vi "VgSweep_TdepRoshan.vi"() -> ()   [LabVIEW 2013]
panel:
  out "Experiment ends at:":string
  in  "How many\npoints:":i16=10 min=-4 max=4 step=1
  in  "Step (K):":dbl=10.0 min=-4.0 max=4.0 step=1.0
  in  "T dependence:":T1(radio)
  in  "Optional custom folder":string
  out "Sweep":i16
  out "T Array":dbl[](array[numeric])
  out "minutes":dbl caption="Last full sweep took:" format="%#.1g"
  in  "Faster":dbl=10.0
  in  "HigherRate?":bool
  out "Current T (K)":dbl min=-4.0 max=4.0 step=0.1 format="%.2f"
  out "T-control\nGPIB":string="24"
  out "Hours":dbl format="%.1f"
  in  "Start sweeping":bool
  out "Of":i16
  out "Estimated time of experiment:":i16
  in  "Sweeps at each T:":i16=1 min=-4 max=4 step=1
  in  "Final T (K)":dbl=145.0 min=-4.0 max=4.0 step=0.1 format="%.2f"
  in  "Initial T (K)":dbl=125.0 min=-4.0 max=4.0 step=0.1 format="%.2f"
  in  "V2:":dbl=1.0 min=-4.0 max=4.0 step=0.1 format="%.3f"
  in  "Sweep rate , V/min":dbl=0.6 min=0.0 max=1.0 step=0.01 format="%.4f"
  in  "V1:":dbl min=-4.0 max=4.0 step=0.1 format="%.3f"
  # "Define interval of gate voltage\nfor main Keithley 2400 (address 12):"
  # "Set temperatures at which sweeps\nare made"
  # "min."
  # "="
  # "hours"
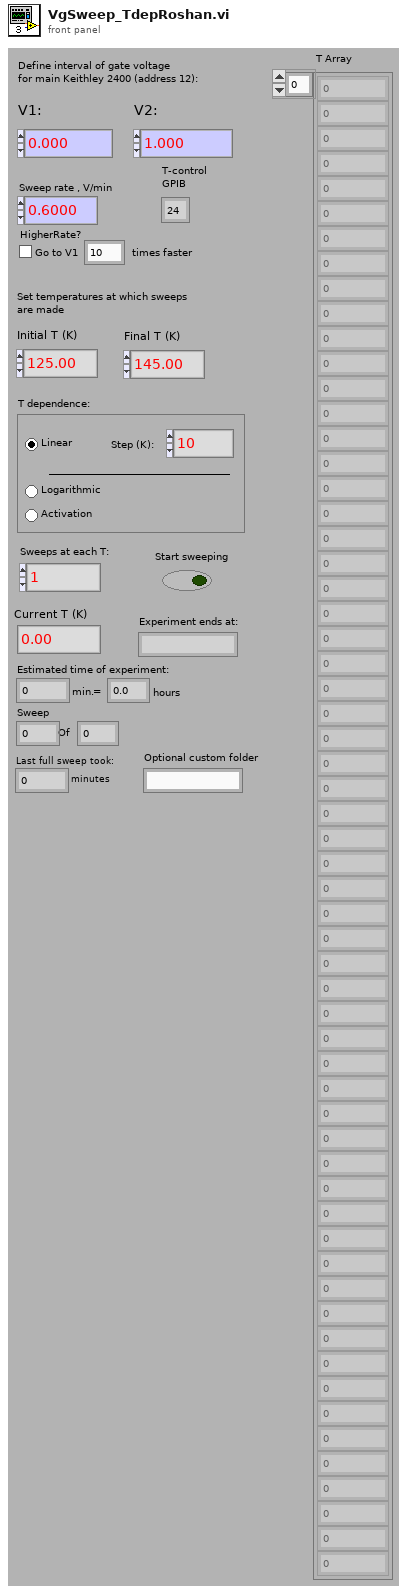
[diagram p1: front panel]
types:
  T1 = enum32{"Radio Selection 1", "Radio Selection 2", "Radio Selection 3"}
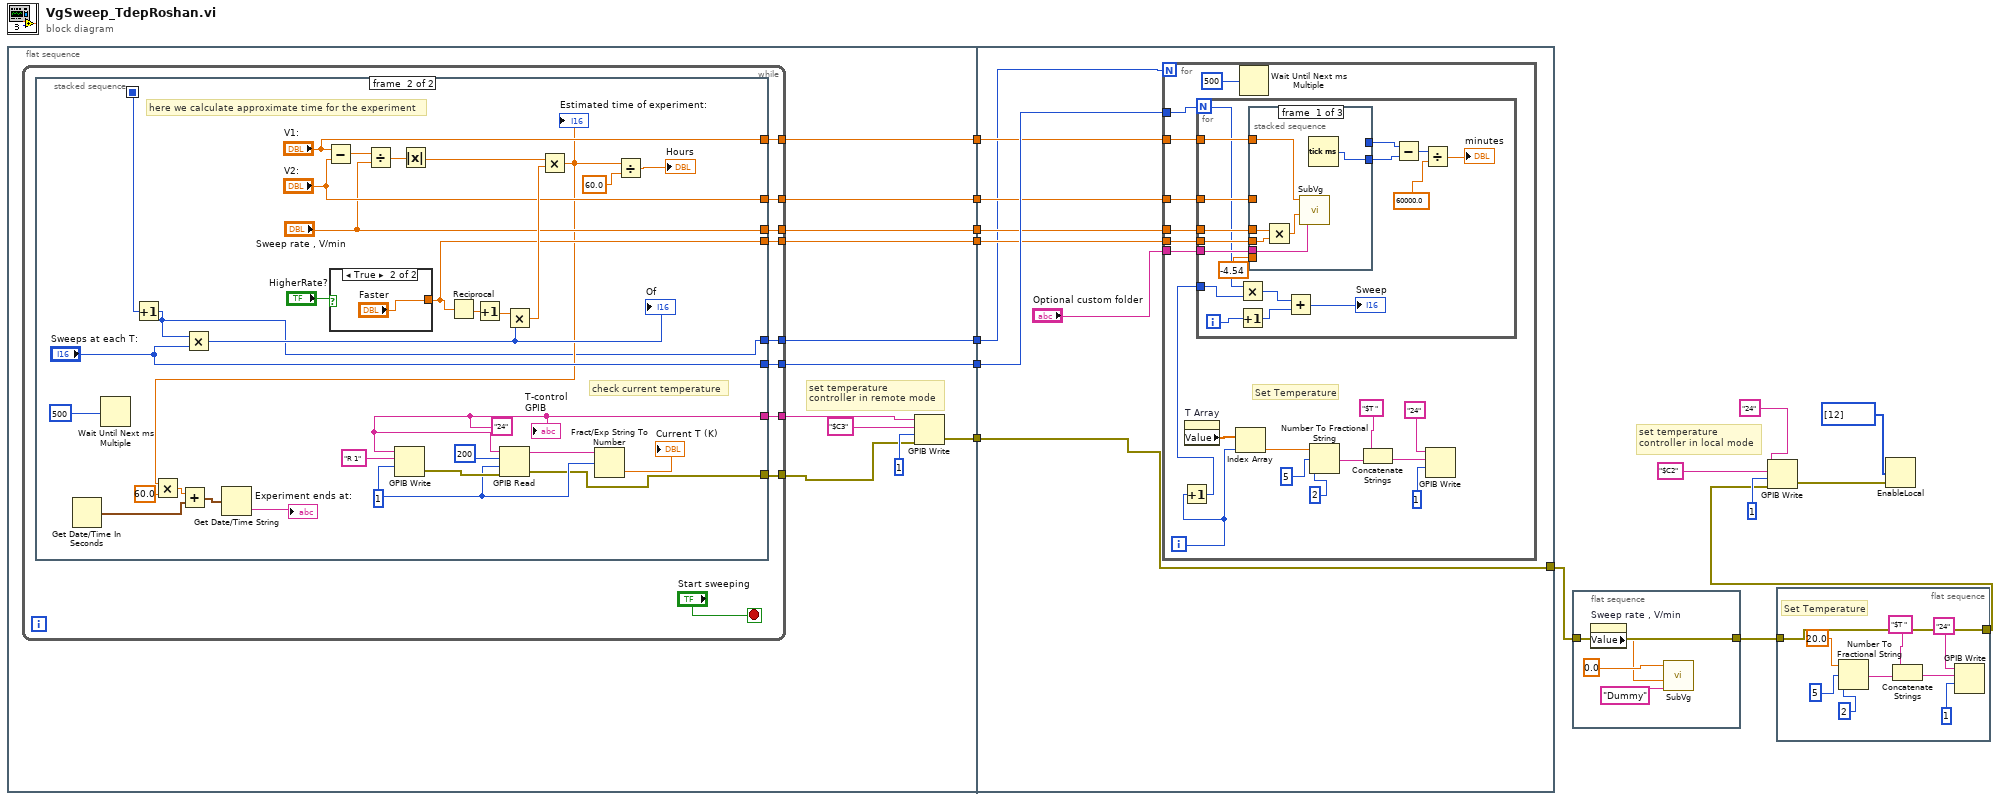
[diagram p0: block diagram]
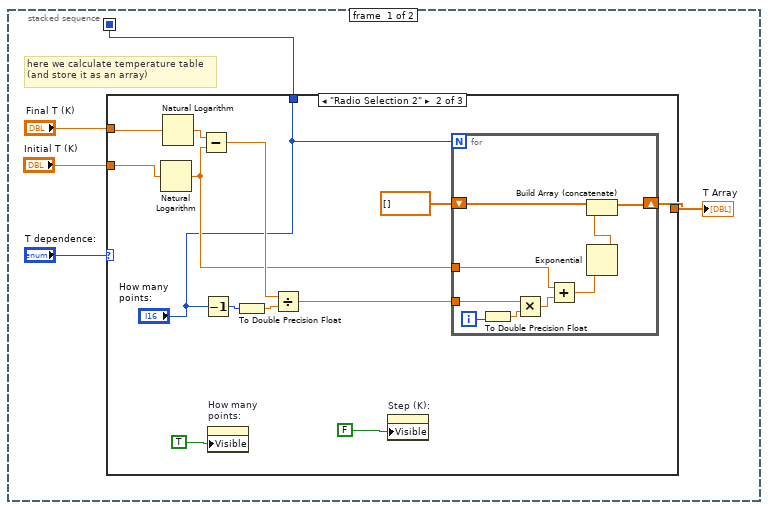
[diagram p2: hidden frame]
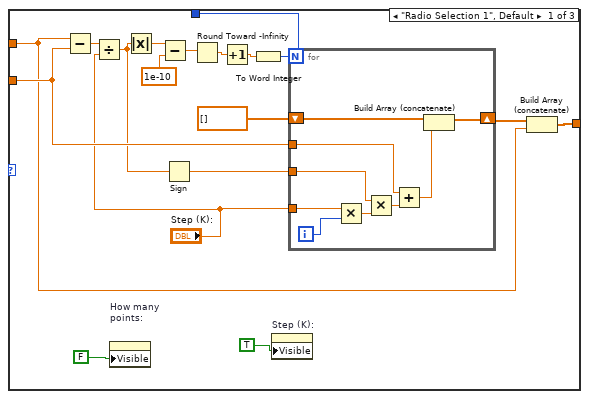
[diagram p3: hidden frame]
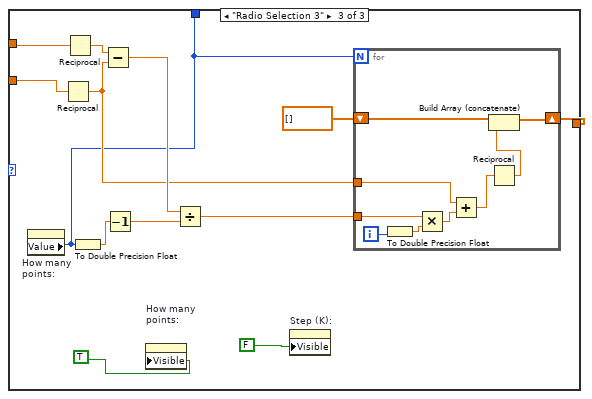
[diagram p4: hidden frame]
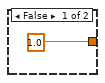
[diagram p5: hidden frame]
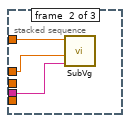
[diagram p6: hidden frame]
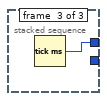
[diagram p7: hidden frame]
diagram:
  # "set temperature\ncontroller in local mode"
  n1 = flat-sequence {
    tunnel: [w24] -> w15
    tunnel: [w23] -> w14
    tunnel: [w22] -> w13
    tunnel: [w21] -> w12
    tunnel: [w20] -> w11
    tunnel: [w19] -> w10
    tunnel: [w17] -> w7
    tunnel: w15 -> [w152]
    tunnel: w14 -> [w151]
    tunnel: w13 -> [w150]
    tunnel: w12 -> [w149]
    tunnel: w11 -> [w148]
    tunnel: w10 -> [w147]
    tunnel: [w146] -> w3
    tunnel: w7 -> [w146]
    frame #0 {
      # "set temperature\ncontroller in remote mode"
      n2 = while {
        tunnel: [w34] -> w16
        tunnel: [w33] -> w18
        tunnel: [w32] -> w24
        tunnel: [w31] -> w23
        tunnel: [w30] -> w22
        tunnel: [w29] -> w21
        tunnel: [w28] -> w20
        tunnel: [w27] -> w19
        stop <- "Start sweeping" stop-if-true
        n3 = stacked-sequence {
          seq-local: [w37 _] -> [_ w120]
          tunnel: [_ w130] -> w34
          tunnel: [_ w118] -> w33
          tunnel: [_ "Sweeps at each T:"] -> w32
          tunnel: [_ "V1:"] -> w31
          tunnel: [_ "V2:"] -> w30
          tunnel: [_ "Sweep rate , V/min"] -> w29
          tunnel: [_ w121] -> w28
          tunnel: [_ w111] -> w27
          frame #0 {
            # "here we calculate temperature table\n(and store it as an array)"
            n4 = case shown="\"Radio Selection 2\"" "T dependence:" {
              tunnel: "Initial T (K)" -> [w52 w76 w99]
              tunnel: [w50 w67 w89] -> w39
              tunnel: "Final T (K)" -> [w49 w77 w100]
              tunnel: [w43 "How many\npoints:" w90] -> w37
              frame "Radio Selection 1", Default {
                n5 = Subtract(x=w49, y=w52) -> (x-y=w47:dbl)
                n6 = Divide(x=w47, y="Step (K):") -> (x/y=w46:dbl)
                n7 = property on="How many\npoints:" class="DigNum (strict)"("Visible"=FALSE) -> ()  [unwired: 2 in, 2 out]
                n8 = Absolute Value(x=w46) -> (abs(x)=w56:dbl)
                n9 = Subtract(x=w56, y=1e-10) -> (x-y=w54:dbl)
                n10 = Sign(1:w46) -> (0:w53:dbl)
                n11 = Round Toward -Infinity(1:w54) -> (0:w48:dbl)
                n12 = Increment(x=w48) -> (x+1=w44:dbl)
                n13 = To Word Integer(number=w44) -> (16bit integer=w43:i16)
                n14 = property on="Step (K):" class="DigNum (strict)"("Visible"=TRUE) -> ()  [unwired: 2 in, 2 out]
                n15 = for {
                  N: w43 -> [_]
                  shift-right: [w58] -> w51
                  shift-left: dbl[] [] -> [w66]
                  tunnel: "Step (K):" -> [w64]
                  tunnel: w53 -> [w62]
                  tunnel: w52 -> [w60]
                  i -> [w63]
                  n16 = Multiply(x=w64, y=w63) -> (x*y=w65:dbl)
                  n17 = Multiply(x=w62, y=w65) -> (x*y=w61:dbl)
                  n18 = Add(x=w60, y=w61) -> (x+y=w59:dbl)
                  n19 = Build Array (concatenate)(w66, w59) -> (w58:dbl[])
                }
                n20 = Build Array (concatenate)(w51, w49) -> (w50:dbl[])
              }
              frame "Radio Selection 2" {
                n21 = Natural Logarithm(1:w76) -> (0:w71:dbl)
                n22 = Natural Logarithm(1:w77) -> (0:w75:dbl)
                n23 = Subtract(x=w75, y=w71) -> (x-y=w74:dbl)
                n24 = Decrement(x="How many\npoints:") -> (x-1=w73:i16)
                n25 = property on="How many\npoints:" class="DigNum (strict)"("Visible"=TRUE) -> ()  [unwired: 2 in, 2 out]
                n26 = To Double Precision Float(number=w73) -> (double precision float=w68:dbl)
                n27 = Divide(x=w74, y=w68) -> (x/y=w72:dbl)
                n28 = property on="Step (K):" class="DigNum (strict)"("Visible"=FALSE) -> ()  [unwired: 2 in, 2 out]
                n29 = for {
                  N: "How many\npoints:" -> [_]
                  shift-right: [w87] -> w67
                  shift-left: dbl[] [] -> [w88]
                  tunnel: w72 -> [w84]
                  tunnel: w71 -> [w82]
                  i -> [w86]
                  n30 = To Double Precision Float(number=w86) -> (double precision float=w85:dbl)
                  n31 = Multiply(x=w84, y=w85) -> (x*y=w83:dbl)
                  n32 = Add(x=w82, y=w83) -> (x+y=w81:dbl)
                  n33 = Exponential(1:w81) -> (0:w80:dbl)
                  n34 = Build Array (concatenate)(w88, w80) -> (w87:dbl[])
                }
              }
              frame "Radio Selection 3" {
                n35 = property on="How many\npoints:" class="DigNum (strict)"() -> ("Value"=w90:i16)  [unwired: 2 in, 2 out]
                n36 = Reciprocal(x=w99) -> (1/x=w94:dbl)
                n37 = Reciprocal(x=w100) -> (1/x=w98:dbl)
                n38 = To Double Precision Float(number=w90) -> (double precision float=w91:dbl)
                n39 = Subtract(x=w98, y=w94) -> (x-y=w97:dbl)
                n40 = Decrement(x=w91) -> (x-1=w96:dbl)
                n41 = property on="How many\npoints:" class="DigNum (strict)"("Visible"=TRUE) -> ()  [unwired: 2 in, 2 out]
                n42 = Divide(x=w97, y=w96) -> (x/y=w95:dbl)
                n43 = property on="Step (K):" class="DigNum (strict)"("Visible"=FALSE) -> ()  [unwired: 2 in, 2 out]
                n44 = for {
                  N: w90 -> [_]
                  shift-right: [w109] -> w89
                  shift-left: dbl[] [] -> [w110]
                  tunnel: w95 -> [w106]
                  tunnel: w94 -> [w104]
                  i -> [w108]
                  n45 = To Double Precision Float(number=w108) -> (double precision float=w107:dbl)
                  n46 = Multiply(x=w106, y=w107) -> (x*y=w105:dbl)
                  n47 = Add(x=w104, y=w105) -> (x+y=w103:dbl)
                  n48 = Reciprocal(x=w103) -> (1/x=w102:dbl)
                  n49 = Build Array (concatenate)(w110, w102) -> (w109:dbl[])
                }
              }
            }
            "T Array" <- w39
          }
          frame #1 {
            w118 = "24"
            w134 = 1
            # "check current temperature"
            # "here we calculate approximate time for the experiment"
            n50 = Get Date/Time In Seconds() -> (seconds since 1Jan1904=w115:timestamp)
            n51 = Wait Until Next ms Multiple(millisecond multiple=500) -> ()  [unwired: 1 out]
            n52 = Increment(x=w120) -> (x+1=w111:i16)
            n53 = Multiply(x=w111, y="Sweeps at each T:") -> (x*y=w119:i16)
            "Of" <- w119
            n54 = Subtract(x="V1:", y="V2:") -> (x-y=w142:dbl)
            n55 = case shown="True" "HigherRate?" {
              tunnel: [1.0 "Faster"] -> w121
              frame False {
              }
              frame True {
              }
            }
            n56 = Divide(x=w142, y="Sweep rate , V/min") -> (x/y=w141:dbl)
            n57 = GPIB Write(0:w118, 1:"R 1", 2:w134) -> (6:w135:errorcluster)  [unwired: 2 in, 1 out]
            n58 = Absolute Value(x=w141) -> (abs(x)=w140:dbl)
            n59 = Reciprocal(x=w121) -> (1/x=w123:dbl)
            n60 = Increment(x=w123) -> (x+1=w127:dbl)
            n61 = GPIB Read(0:w118, 1:200, 2:w134, 3:w135) -> (5:w136:string, 7:w130:errorcluster)  [unwired: 1 in, 1 out]
            n62 = Multiply(x=w127, y=w119) -> (x*y=w129:dbl)
            n63 = Multiply(x=w140, y=w129) -> (x*y=w112:dbl)
            "Estimated time of experiment:" <- w112
            n64 = Multiply(x=w112, y=60.0) -> (x*y=w116:dbl)
            n65 = Add(x=w116, y=w115) -> (x+y=w114:timestamp)
            n66 = Get Date/Time String(seconds (now)=w114) -> (time string=→"Experiment ends at:":string)  [unwired: 2 in, 1 out]
            n67 = Fract/Exp String To Number(string=w136, offset=w134) -> (number=→"Current T (K)":dbl)  [unwired: 2 in, 1 out]
            n68 = Divide(x=w112, y=60.0) -> (x/y=→"Hours":dbl)
            "T-control\nGPIB" <- w118
          }
        }
      }
      n69 = GPIB Write(0:w18, 1:"$C3", 2:1, 3:w16) -> (6:w17:errorcluster)  [unwired: 1 in, 1 out]
    }
    frame #1 {
      n70 = for {
        N: w147 -> [_]
        tunnel: w152 -> [w163]
        tunnel: w151 -> [w162]
        tunnel: w150 -> [w161]
        tunnel: w149 -> [w160]
        tunnel: w148 -> [w159]
        tunnel: "Optional custom folder" -> [w154]
        i -> [w157]
        # "Set Temperature"
        n71 = Increment(x=w157) -> (x+1=w153:i32)
        n72 = property on="T Array" class="Arr (strict)"() -> ("Value"=w165:dbl[])  [unwired: 2 in, 2 out]
        n73 = for {
          N: w163 -> [w176]
          tunnel: w162 -> [w185]
          tunnel: w161 -> [w187]
          tunnel: w160 -> [w186]
          tunnel: w159 -> [w184]
          tunnel: w154 -> [w178]
          tunnel: w153 -> [w175]
          i -> [w177]
          n74 = Multiply(x=w176, y=w175) -> (x*y=w174:i32)
          n75 = Increment(x=w177) -> (x+1=w173:i32)
          n76 = stacked-sequence {
            tunnel: w187 -> [_ w196 _]
            tunnel: w186 -> [w192 w195 _]
            tunnel: w185 -> [w193 _ _]
            tunnel: w184 -> [w191 _ _]
            tunnel: [w189 _ _] -> w180
            tunnel: [_ _ w197] -> w179
            tunnel: w178 -> [w188 w194 _]
            tunnel: -4.54 -> [_ _ _]
            frame #0 {
              n77 = Multiply(x=w192, y=w191) -> (x*y=w190:dbl)
              n78 = call "SubVg.vi"("Target Voltage, V"=w193, "Sweep rate, V/min"=w190, "Custom Folder"=w188) -> ()  [unwired: 7 in]
              n79 = Tick Count (ms)() -> (millisecond timer value=w189:u32)
            }
            frame #1 {
              n80 = call "SubVg.vi"("Target Voltage, V"=w196, "Sweep rate, V/min"=w195, "Custom Folder"=w194) -> ()  [unwired: 7 in]
            }
            frame #2 {
              n81 = Tick Count (ms)() -> (millisecond timer value=w197:u32)
            }
          }
          n82 = Add(x=w174, y=w173) -> (x+y=→"Sweep":i32)
          n83 = Subtract(x=w179, y=w180) -> (x-y=w183:u32)
          n84 = Divide(x=w183, y=60000.0) -> (x/y=→"minutes":dbl)
        }
        n85 = Index Array(array=w165, index=w157) -> (element=w164:dbl)
        n86 = Wait Until Next ms Multiple(millisecond multiple=500) -> ()  [unwired: 1 out]
        n87 = Number To Fractional String(number=w164, width (-)=5, precision (6)=2) -> (F-format string=w167:string)  [unwired: 1 in]
        n88 = Concatenate Strings("$T ", w167) -> (w166:string)
        n89 = GPIB Write(0:"24", 1:w166, 2:1) -> ()  [unwired: 2 in, 2 out]
      }
    }
  }
  n90 = flat-sequence {
    tunnel: w3 -> [w201]
    tunnel: [w201] -> w2
    frame #0 {
      n91 = property on="Sweep rate , V/min" class="DigNum (strict)"() -> ("Value"=w198:dbl)  [unwired: 2 in, 2 out]
      n92 = call "SubVg.vi"("Target Voltage, V"=0.0, "Sweep rate, V/min"=w198, "Custom Folder"="Dummy") -> ()  [unwired: 7 in]
    }
  }
  n93 = GPIB Write(0:"24", 1:"$C2", 2:1, 3:w1) -> (6:w4:errorcluster)  [unwired: 1 in, 1 out]
  n94 = flat-sequence {
    tunnel: w2 -> [w202]
    tunnel: [w202] -> _
    tunnel: [w202] -> w1
    frame #0 {
      # "Set Temperature"
      n95 = Number To Fractional String(number=20.0, width (-)=5, precision (6)=2) -> (F-format string=w206:string)  [unwired: 1 in]
      n96 = Concatenate Strings("$T ", w206) -> (w207:string)
      n97 = GPIB Write(0:"24", 1:w207, 2:1) -> ()  [unwired: 2 in, 2 out]
    }
  }
  n98 = EnableLocal(2:w4, 3:i32[] [12]) -> ()  [unwired: 1 in, 2 out]
